vi "test Verify CLI Echo Hello World.vi"(8 "error in":errorcluster, 11 "Test Case In":refnum<class "LUnit Extensions Tests.lvclass">) -> (0 "error out":errorcluster, 3 "Test Case Out":refnum<class "LUnit Extensions Tests.lvclass">)   [LabVIEW 2020, in "LUnit Extensions Tests.lvclass"]
uses:
  LUnit Extensions Tests.lvclass
  C:/Program Files/National Instruments/LabVIEW 2026/vi.lib/Astemes/LUnit/Test Case.lvclass
  Source/Extensions/LUnit.Extension/LUnit.Extension.lvlib
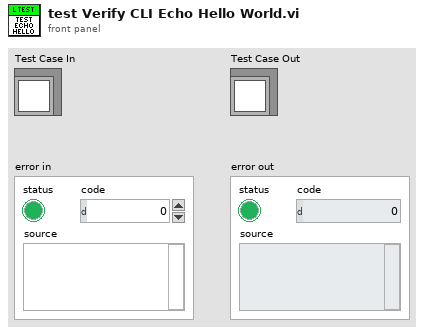
[diagram p1: front panel]
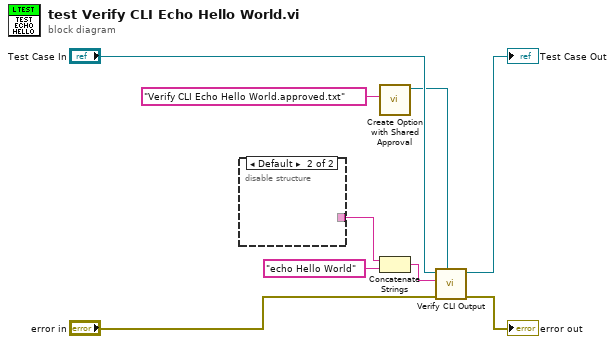
[diagram p0: block diagram]
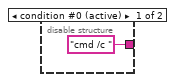
[diagram p2: hidden frame]
diagram:
  n1 = disable-structure shown="Default" {
    disable-tunnel: ["cmd /c " _] -> w5
    frame condition #0 (active) {
    }
    frame condition #1 {
    }
  }
  n2 = call "Create Option with Shared Approval.vi"("Filename"="Verify CLI Echo Hello World.approved.txt") -> ("Options outs"=w1:refnum<class "Options.lvclass">)  [unwired: 10 in]
  n3 = Concatenate Strings(w5, "echo Hello World" ("command line")) -> (w3:string)
  n4 = call "Verify CLI Output.vi"("Options"=w1, "error in"="error in", "command line"=w3, "LUnit Test Case In"="Test Case In") -> ("error out"=→"error out":errorcluster, "LUnit Test Case Out"=→"Test Case Out":refnum<class "LUnit Extensions Tests.lvclass">)  [unwired: 6 in]
